vi "TCP Initiate.vi"(11 "IP ADDRESS":string="192.168.3.250") -> (0 "error out":errorcluster, 3 "connection ID":refnum<k5>)   [LabVIEW 2023]
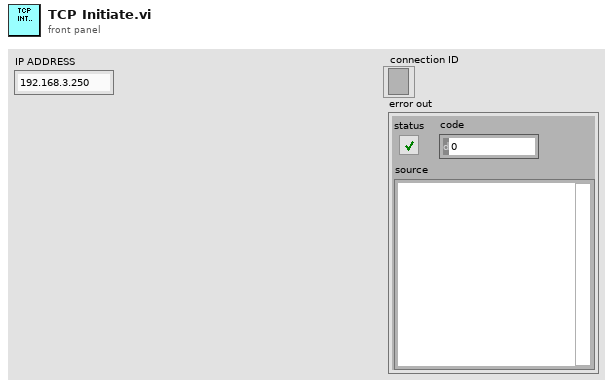
[diagram p1: front panel]
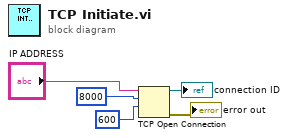
[diagram p0: block diagram]
diagram:
  n1 = TCP Open Connection(address="IP ADDRESS", remote port or service name=u16 8000 ("remote port"), timeout ms (60000)=600) -> (connection ID=→"connection ID":refnum<k5>, error out=→"error out":errorcluster)  [unwired: 2 in]
